vi "lockin - add phase element.vi"(8 "error in (no error)":errorcluster, 11 "Lockin.DAQ":refnum<class "Lockin.DAQ.lvclass">) -> (0 "error out":errorcluster, 3 "Lockin.DAQ out":refnum<class "Lockin.DAQ.lvclass">)   [LabVIEW 2019]
uses:
  Lockin.DAQ.lvclass
  C:/Program Files (x86)/National Instruments/LabVIEW 2016/vi.lib/JKI/JKI SMO/SMO/SMO.lvclass
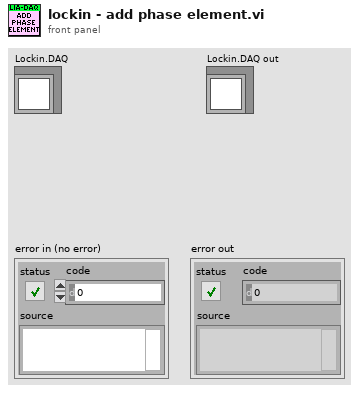
[diagram p1: front panel]
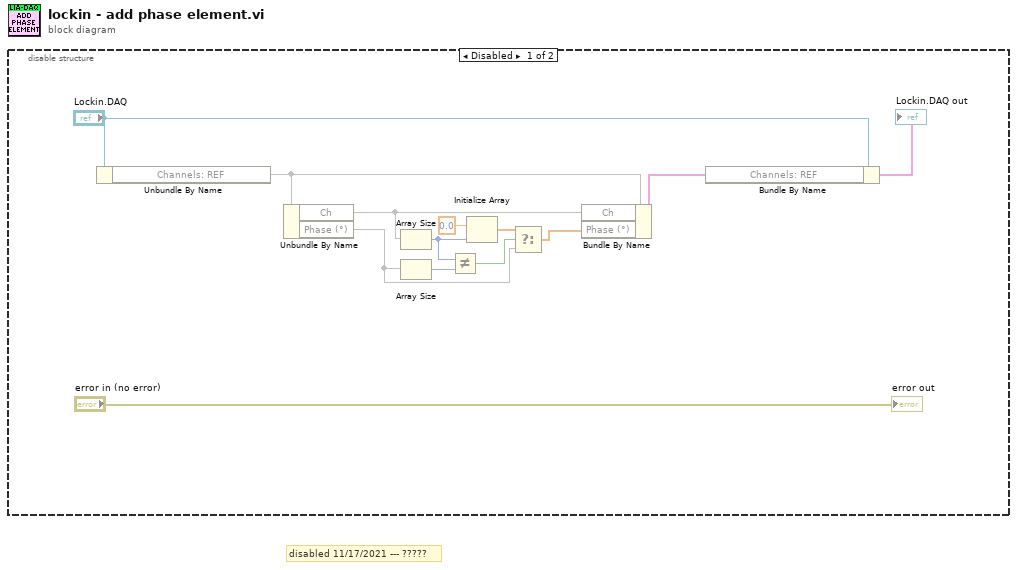
[diagram p0: block diagram]
diagram:
  # "disabled 11/17/2021 --- ?????"
  n1 = disable-structure shown="Disabled" {
    frame Disabled {
      n2 = Unbundle By Name("Lockin.DAQ") -> ("Channels: REF"=w3)
      n3 = Unbundle By Name(w3) -> ("Ch"=w11, "Phase (°)"=w9)
      n4 = Array Size(array=w11) -> (size(s)=w6:i32)
      n5 = Array Size(array=w9) -> (size(s)=w12:i32)
      n6 = Not Equal?(x=w6, y=w12) -> (x != y?=w13:bool)
      n7 = Initialize Array(0.0 ("element"), w6) -> (w8:dbl[])
      n8 = Select(t=w8, s=w13, f=w9) -> (s? t:f=w10:dbl[])
      n9 = Bundle By Name(cluster=w3, "Ch"=w11, "Phase (°)"=w10) -> (w1:cluster{})
      n10 = Bundle By Name(cluster="Lockin.DAQ", "Channels: REF"=w1) -> (→"Lockin.DAQ out":cluster{})
      "error out" <- "error in (no error)"
    }
    frame Enabled {
    }
  }
